vi "OA Add Mode.vi"(7 "uiModeDescriptionLen":u32, 9 "pcModeDescription":string, 10 "uiModeNameLen":u32, 11 "pcModeName":string) -> (1 "pcModeDescription out":string, 2 "function return":u32, 3 "pcModeName out":string)   [LabVIEW 2018, in "AndorSDK.lvlib"]
doc: "EXPNETTYPE unsigned int WINAPI OA_AddMode(char * pcModeName, unsigned int uiModeNameLen, char * pcModeDescription, unsigned int uiModeDescriptionLen);"
uses:
  AndorSDK.lvlib
  ATMCD32D.dll
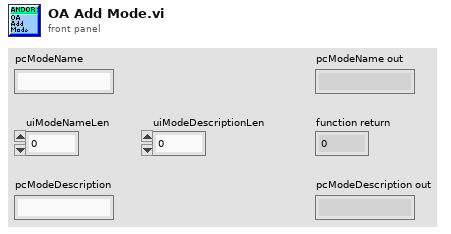
[diagram p1: front panel]
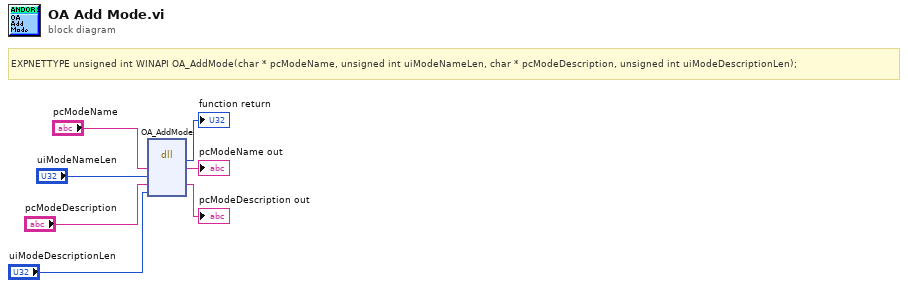
[diagram p0: block diagram]
diagram:
  # "EXPNETTYPE unsigned int WINAPI OA_AddMode(char * pcModeName, unsigned int uiModeNameLen, char * pcModeDescription, unsigned int uiModeDescriptionLen);"
  n1 = dll-call lib="PTH2babs E\nPersönliches02 - Arbeit03-HiwijobsLabviewCodelibANDOR\tAndor SDK\nATMCD32D.*" fn="OA_AddMode"("pcModeName"="pcModeName", "uiModeNameLen"="uiModeNameLen", "pcModeDescription"="pcModeDescription", "uiModeDescriptionLen"="uiModeDescriptionLen") -> (→"function return":u32, "pcModeName"=→"pcModeName out":string, "pcModeDescription"=→"pcModeDescription out":string)  [unwired: 5 in, 2 out]
